vi "EventServer_GetClientSubscriptions.vi"(8 "error in (no error)":errorcluster, 11 "Client Name":string) -> (0 "error out":errorcluster, 3 "Subscription":string[](array[string]))   [LabVIEW 2011]
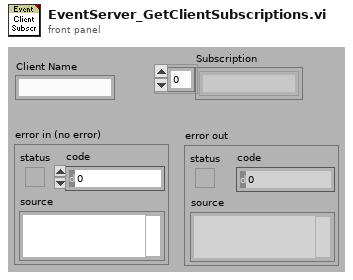
[diagram p1: front panel]
types:
  T1 = cluster{"Client":refnum<queue>, "Sub Events":string[], "PrvData":variant, "MyName":string}
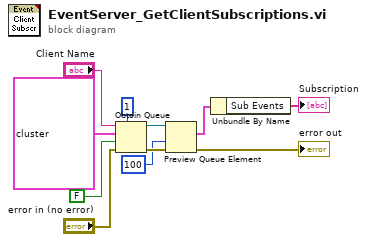
[diagram p0: block diagram]
diagram:
  n1 = Obtain Queue(max queue size (-1, unlimited)=1, name (unnamed)="Client Name", element data type=T1 {"Client"=refnum, "Sub Events"=[], "PrvData"=variant, "MyName"=""} ("output cluster"), create if not found? (T)=FALSE, error in (no error)="error in (no error)") -> (queue out=w7:refnum<queue>, error out=w6:errorcluster)  [unwired: 1 out]
  n2 = Preview Queue Element(queue=w7, timeout in ms (-1)=100, error in (no error)=w6) -> (element=w5:T1, error out=→"error out":errorcluster)  [unwired: 2 out]
  n3 = Unbundle By Name(w5) -> ("Sub Events"=→"Subscription":string[])
